vi "Calculadora_b.vi"() -> ()   [LabVIEW 2019]
panel:
  out "Resultado":dbl
  in  "Division":bool
  in  "Resta":bool
  in  "Multiplicacion":bool
  in  "Suma":bool
  in  "Numero 2":dbl
  in  "Numero 1":dbl
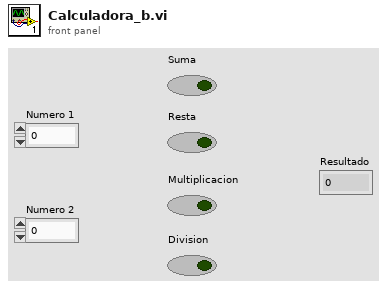
[diagram p1: front panel]
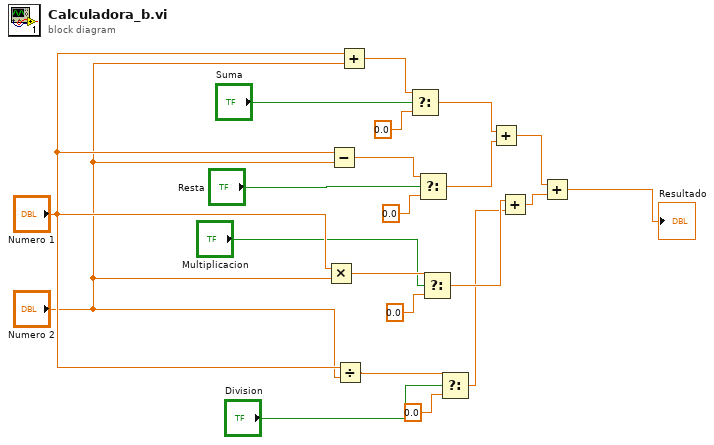
[diagram p0: block diagram]
diagram:
  n1 = Multiply(x="Numero 1", y="Numero 2") -> (x*y=w15:dbl)
  n2 = Subtract(x="Numero 1", y="Numero 2") -> (x-y=w16:dbl)
  n3 = Divide(x="Numero 1", y="Numero 2") -> (x/y=w11:dbl)
  n4 = Add(x="Numero 1", y="Numero 2") -> (x+y=w8:dbl)
  n5 = Select(t=w8, s="Suma", f=0.0) -> (s? t:f=w7:dbl)
  n6 = Select(t=w16, s="Resta", f=0.0) -> (s? t:f=w6:dbl)
  n7 = Select(t=w15, s="Multiplicacion", f=0.0) -> (s? t:f=w5:dbl)
  n8 = Select(t=w11, s="Division", f=0.0) -> (s? t:f=w4:dbl)
  n9 = Add(x=w7, y=w6) -> (x+y=w3:dbl)
  n10 = Add(x=w5, y=w4) -> (x+y=w2:dbl)
  n11 = Add(x=w3, y=w2) -> (x+y=→"Resultado":dbl)
